vi "Test Timed Flush.vi"(8 "error in":errorcluster) -> (0 "error out":errorcluster)   [LabVIEW 2016, in "UT_FileHandler.lvlib"]
doc: "Test the processing of an LogRecord."
uses:
  UT_FileHandler.lvlib
  Source/HSE-Logger/LogLevel.ctl
  <vilib>/addons/_JKI Toolkits/Caraya/classes/Assert/Assert Equal Value_Variant.vi
  Source/HSE-Logger/Handler/FileHandler/FileHandler.lvclass
  <vilib>/addons/_JKI Toolkits/Caraya/classes/Test/Test.lvclass
  Source/HSE-Logger/hse-logger.lvlib
  Source/HSE-Logger/LogRecord/LogRecord.lvclass
  <vilib>/addons/_JKI Toolkits/Caraya/classes/Assert/Assert.lvclass
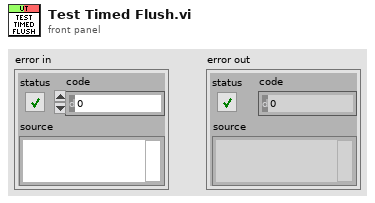
[diagram p1: front panel]
types:
  T1 = typedef "hse-logger.lvlib/LogLevel.ctl" = enum16{"DEBUG", "INFO", "WARNING", "ERROR", "CRITICAL"}
  T2 = enum16{"open", "replace", "create", "open or create", "replace or create", "replace or create with confirmation"}
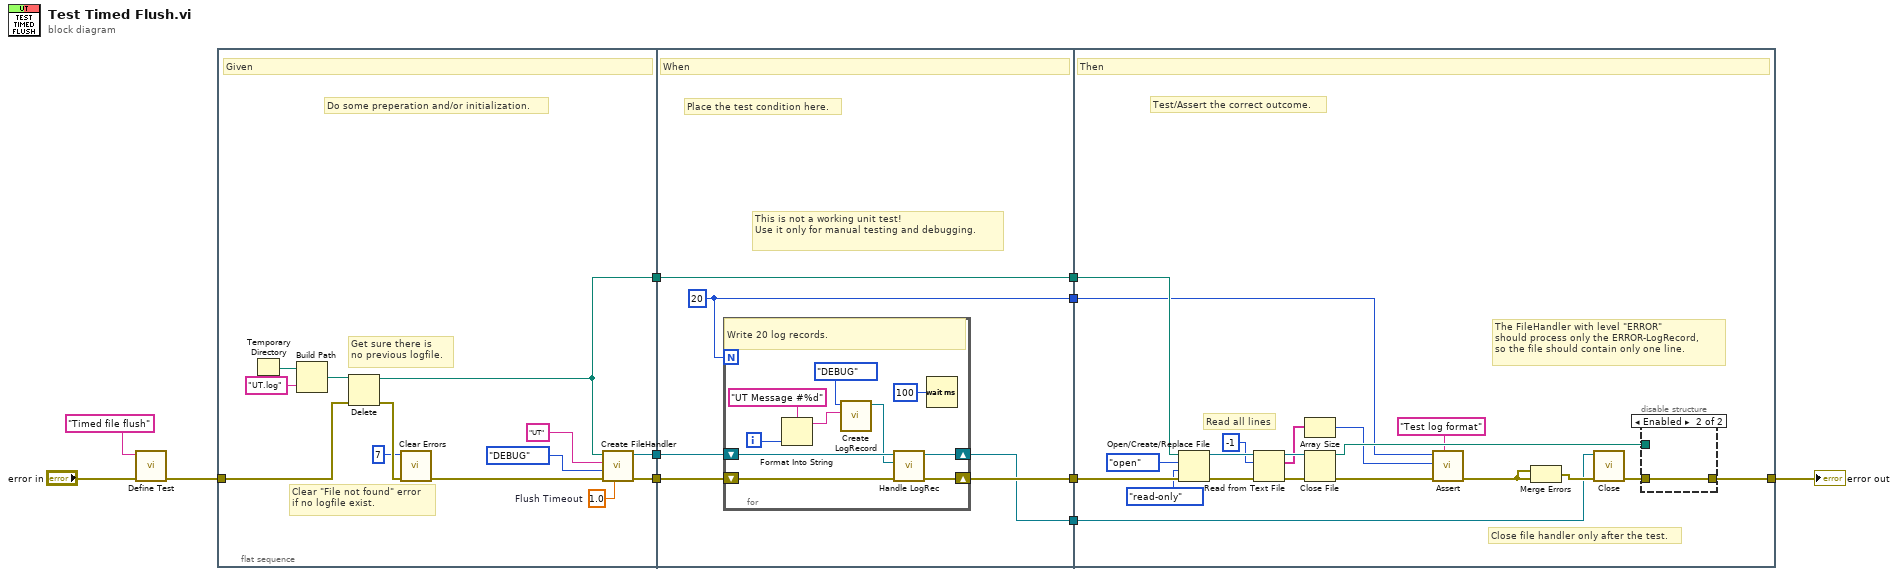
[diagram p0: block diagram]
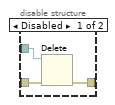
[diagram p2: hidden frame]
diagram:
  n1 = call <vilib>:"Define Test.vi"("error in (no error)"="error in", "Label (VI Title)"="Timed file flush") -> ("error out"=w8:errorcluster)  [unwired: 8 in, 1 out]
  n2 = flat-sequence {
    tunnel: w8 -> [w24]
    tunnel: [w22] -> w11
    tunnel: [w16] -> w5
    tunnel: [w14] -> w3
    tunnel: w11 -> [w29]
    tunnel: [w30] -> w7
    tunnel: w5 -> [w27]
    tunnel: [w27] -> w4
    tunnel: w3 -> [w28]
    tunnel: [w26] -> w2
    tunnel: [w25] -> w1
    tunnel: [w57] -> w10
    tunnel: w7 -> [w60]
    tunnel: w4 -> [w52]
    tunnel: w2 -> [w44]
    tunnel: w1 -> [w42]
    frame #0 {
      w13 = 1.0  # Flush Timeout
      # "Clear \"File not found\" error\nif no logfile exist."
      # "Get sure there is\nno previous logfile."
      # "Do some preperation and/or initialization."
      # "Given"
      n3 = Temporary Directory() -> (w20:path)
      n4 = Build Path(base path=w20, name or relative path="UT.log") -> (appended path=w18:path)
      n5 = Delete(path (use dialog)=w18, error in=w24) -> (deleted path=w16:path, error out=w23:errorcluster)  [unwired: 3 in, 1 out]
      n6 = call <vilib>:"Clear Errors.vi"("error in (no error)"=w23, "specific error code to clear (0: all)"=7) -> ("error out"=w21:errorcluster)  [unwired: 4 in, 1 out]
      n7 = call "Create FileHandler.vi"("Flush Timeout (0 s)"=w13, "error in"=w21, "Level"=LogLevel."DEBUG", "Name"="UT", "Filepath"=w16) -> ("error out"=w22:errorcluster, "FileHandler out"=w14:refnum<class "FileHandler.lvclass">)  [unwired: 5 in]
    }
    frame #1 {
      w25 = 20
      # "This is not a working unit test!\nUse it only for manual testing and debugging."
      # "Place the test condition here."
      # "When"
      n8 = for {
        N: w25 -> [_]
        shift-right: [w35] -> w26
        shift-left: w28 -> [w38]
        shift-right: [w39] -> w30
        shift-left: w29 -> [w40]
        i -> [w33]
        # "Write 20 log records."
        n9 = Format Into String(format string="UT Message #%d" ("Message"), w33) -> (resulting string=w32:string)  [unwired: 2 in, 1 out]
        n10 = call "Create LogRecord.vi"("Message"=w32, "Level"=LogLevel."DEBUG") -> ("LogRecord out"=w36:refnum<class "LogRecord.lvclass">)  [unwired: 8 in, 1 out]
        n11 = call-dynamic "Handle LogRec.vi"("error in"=w40, "LogRecord"=w36, "FileHandler in"=w38) -> ("error out"=w39:errorcluster, "FileHandler out"=w35:refnum<class "FileHandler.lvclass">)  [unwired: 7 in]
        n12 = Wait (ms)(milliseconds to wait=u32 100) -> ()  [unwired: 1 out]
      }
    }
    frame #2 {
      # "Close file handler only after the test."
      # "The FileHandler with level \"ERROR\"\nshould process only the ERROR-LogRecord,\nso the file should contain only one line."
      # "Read all lines"
      # "Test/Assert the correct outcome."
      # "Then"
      n13 = Open/Create/Replace File(file path (use dialog)=w52, error in=w60, operation (0:open)=T2."open", access (0:read/write)=enum16{"read/write", "read-only", "write-only"}."read-only") -> (refnum out=w49:refnum<file>, error out=w59:errorcluster)  [unwired: 2 in, 1 out]
      n14 = Read from Text File(file (use dialog)=w49, count=-1, error in=w59) -> (refnum out=w48:refnum<file>, text=w45:string[], error out=w58:errorcluster)  [unwired: 1 in, 1 out]
      n15 = Array Size(array=w45) -> (size(s)=w43:i32)
      n16 = Close File(refnum=w48, error in=w58) -> (path=w47:path, error out=w54:errorcluster)
      n17 = call-poly <vilib>:"Assert.vi"("Label"="Test log format", "error in (no error)"=w54, "Y"=w43, "X"=w42) -> ("error out"=w53:errorcluster)  [unwired: 6 in, 1 out]
      n18 = Merge Errors(w53, w53) -> (w56:errorcluster)
      n19 = call-dynamic "Close.vi"("error in"=w56, "FileHandler in"=w44) -> ("error out"=w55:errorcluster)  [unwired: 8 in, 1 out]
      n20 = disable-structure shown="Enabled" {
        disable-tunnel: [w63 w64] -> w57
        disable-tunnel: w47 -> [w61 _]
        disable-tunnel: w55 -> [w62 w64]
        frame Disabled {
          n21 = Delete(path (use dialog)=w61, error in=w62) -> (error out=w63:errorcluster)  [unwired: 3 in, 2 out]
        }
        frame Enabled {
        }
      }
    }
  }
  "error out" <- w10
